vi "Module Did Init.vi"(8 "error in":errorcluster, 9 "Initialized?":bool, 10 "Origin":string) -> (0 "error out":errorcluster)   [LabVIEW 2026, in "Acquisition.lvlib"]
doc: "Send the Module Did Init event to any VI registered to listen to this module's broadcast events.\n_____\nBased on DQMH Project Template 4.0.0.47.\n_____\nBased on DQMH Dev Tools: Project Template 7.1.2.1547."
uses:
  Acquisition.lvlib
  Did Init Argument--cluster.ctl
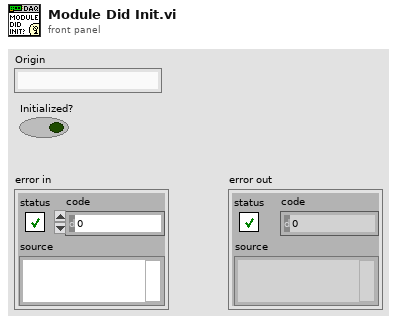
[diagram p1: front panel]
types:
  T1 = typedef "Acquisition.lvlib/Did Init Argument--cluster.ctl" = cluster{"Init?":bool, "Info":string}
  T2 = typedef "Acquisition.lvlib/Broadcast Events--cluster.ctl" = cluster{"Module Did Init":refnum<user-event>, "Status Updated":refnum<user-event>, "Error Reported":refnum<user-event>, "Module Did Stop":refnum<user-event>, "Update Module Execution Status":refnum<user-event>, "Acquisition Started":refnum<user-event>, "Acquisition Stopped":refnum<user-event>, "Data Updated":refnum<user-event>, "Device Calibrated":refnum<user-event>}
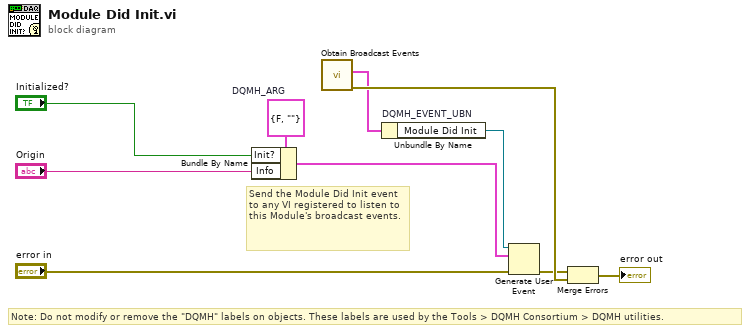
[diagram p0: block diagram]
diagram:
  w2 = T1 {"Init?"=FALSE, "Info"=""}  # DQMH_ARG
  # "Note: Do not modify or remove the \"DQMH\" labels on objects. These labels are used by the Tools > DQMH Consortium > DQMH utilities."
  # "Send the Module Did Init event to any VI registered to listen to this Module's broadcast events."
  n1 = Bundle By Name(cluster=w2, "Init?"="Initialized?", "Info"="Origin") -> (w1:T1)
  n2 = call "Obtain Broadcast Events.vi"() -> ("error out"=w6:errorcluster, "Acquisition Broadcast Events"=w4:T2)  [unwired: 10 in]
  n3 = Unbundle By Name "DQMH_EVENT_UBN"(w4) -> ("Module Did Init"=w3:refnum<user-event>)
  n4 = Generate User Event(user event=w3, event data cluster=w1, error in="error in") -> (error out=w5:errorcluster)  [unwired: 1 in, 1 out]
  n5 = Merge Errors(w5, w6) -> (→"error out":errorcluster)
